vi "CameraAcquireImage.vi"(8 "error in":errorcluster, 10 "cam index":i32, 11 "Index":i32) -> (0 "error out":errorcluster, 4 "return":i32)   [LabVIEW 2019]
uses:
  [Global] CameraSessionArray.vi
  [Global] Image.vi
  <vilib>/vision/driver/NI_Vision_Acquisition_Software.lvlib
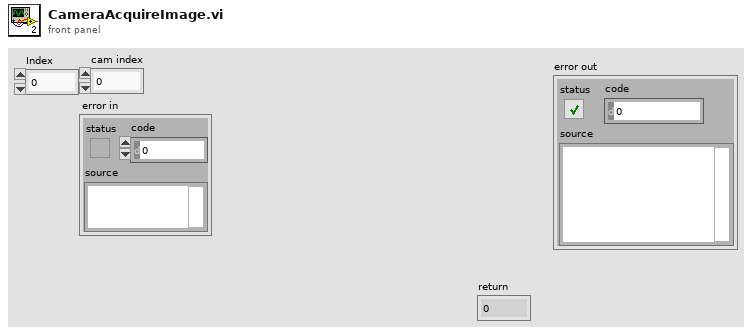
[diagram p1: front panel]
types:
  T1 = typedef "IMAQdx.ctl" = refnum<k21>
  T2 = typedef "IMAQ Image.ctl" = refnum<image>
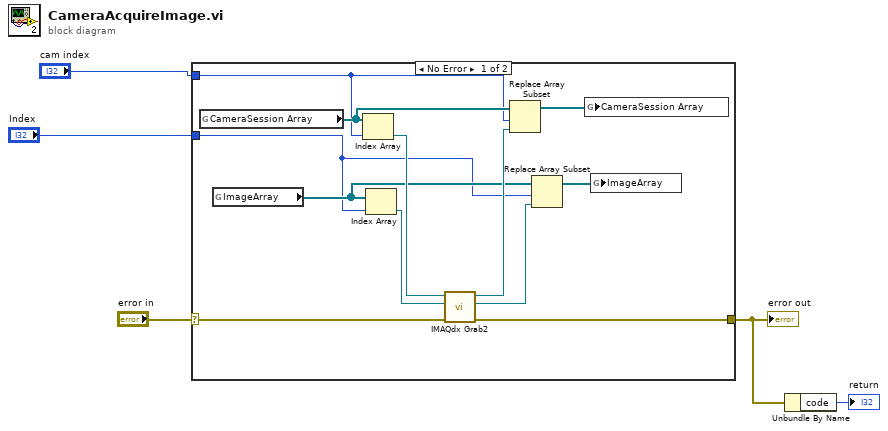
[diagram p0: block diagram]
diagram:
  n1 = case shown="No Error" "error in" {
    selector: "error in" -> [w17 w18]
    tunnel: [w16 w18] -> w3
    tunnel: "Index" -> [w8 _]
    tunnel: "cam index" -> [w6 _]
    frame No Error {
      n2 = global read "[Global] CameraSessionArray.vi" "CameraSession Array"() -> (w13:T1[])
      n3 = global read "[Global] Image.vi" "ImageArray"() -> (w10:T2[])
      n4 = Index Array(array=w13, index=w6) -> (element=w15:T1)
      n5 = Index Array(array=w10, index=w8) -> (element=w14:T2)
      n6 = call <vilib>:"IMAQdx Grab2.vi"("error in"=w17, "Image In"=w14, "Session In"=w15) -> ("error out"=w16:errorcluster, "Image Out"=w9:T2, "Session Out"=w12:T1)  [unwired: 5 in, 1 out]
      n7 = Replace Array Subset(array=w13, new element=w12, index=w6) -> (w11:T1[])
      n8 = Replace Array Subset(array=w10, new element=w9, index=w8) -> (w7:T2[])
      n9 = global write "[Global] CameraSessionArray.vi" "CameraSession Array"(w11) -> ()
      n10 = global write "[Global] Image.vi" "ImageArray"(w7) -> ()
    }
    frame Error {
    }
  }
  "error out" <- w3
  n11 = Unbundle By Name(w3) -> ("code"=→"return":i32)
